vi "Default Settings.vi"(8 "error in (no error)":errorcluster, 10 "Module In":refnum<class "Module.lvclass">, 11 "Component in":refnum<class "Component Tray.lvclass">) -> (0 "error out":errorcluster, 2 "Module Out":refnum<class "Module.lvclass">, 3 "Component out":refnum<class "Component Tray.lvclass">)   [LabVIEW 2020, in "Component Tray.lvclass"]
uses:
  Component Tray.lvclass
  Module/Module.lvclass
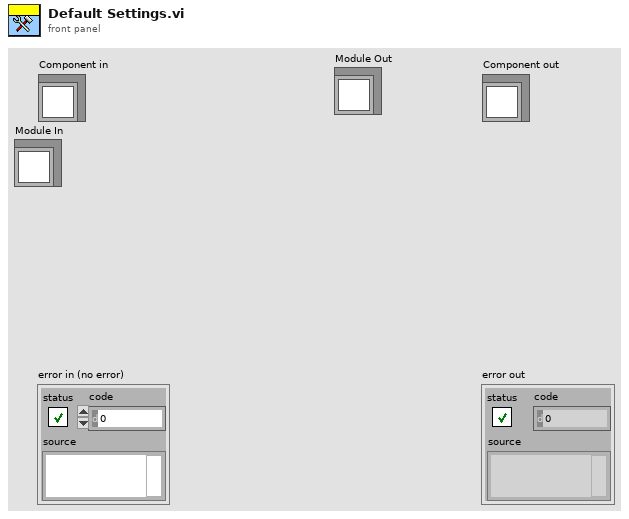
[diagram p1: front panel]
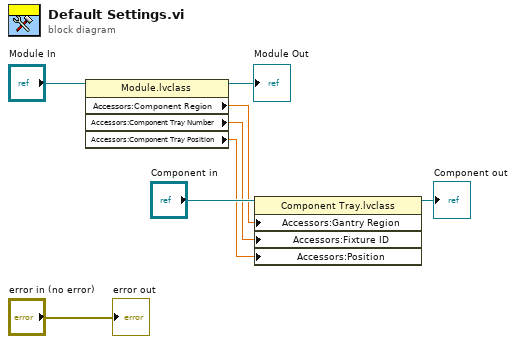
[diagram p0: block diagram]
diagram:
  n1 = property class="Module.lvclass"(reference="Module In") -> (reference out=→"Module Out":refnum<class "Module.lvclass">, "Accessors:Component Region"=w4:dbl, "Accessors:Component Tray Number"=w3:dbl, "Accessors:Component Tray Position"=w2:dbl)  [unwired: 1 in, 1 out]
  n2 = property class="Component Tray.lvclass"(reference="Component in", "Accessors:Gantry Region"=w4, "Accessors:Fixture ID"=w3, "Accessors:Position"=w2) -> (reference out=→"Component out":refnum<class "Component Tray.lvclass">)  [unwired: 1 in, 1 out]
  "error out" <- "error in (no error)"
